vi "3.1.vi"() -> ()   [LabVIEW 2017]
panel:
  out "波形图":dbl[](graph)
  out "平均":dbl
  out "最小":dbl
  out "最大":dbl
  in  "长按停止":bool
  in  "生成随机数":bool
  # "任务一"
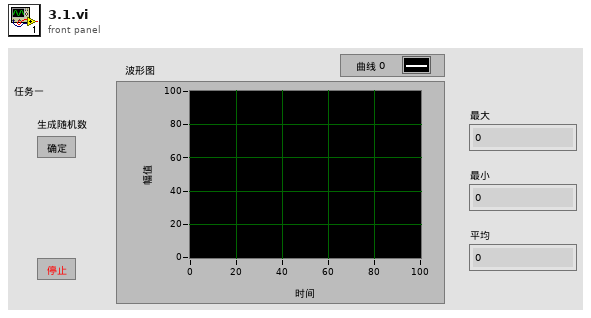
[diagram p1: front panel]
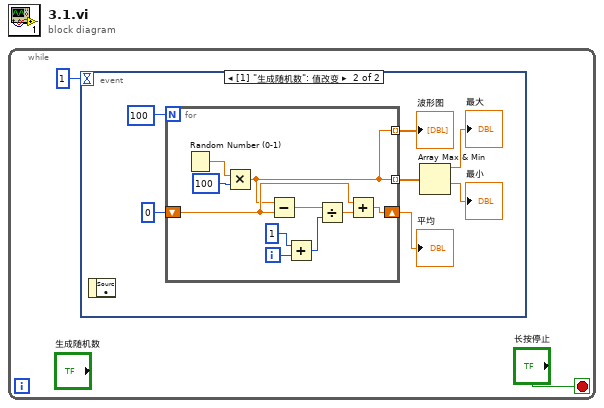
[diagram p0: block diagram]
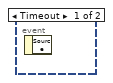
[diagram p2: hidden frame]
diagram:
  n1 = while {
    stop <- "长按停止" stop-if-true
    n2 = event shown="[1] \"生成随机数\": 值改变" {
      selector: _ -> [_ _]
      dyn-events: _ -> [_ _]
      timeout: 1 -> [_ _]
      event Timeout {
        n3 = event-data() -> ()  [unwired: 1 in, 1 out]
      }
      event "生成随机数": Value Change {
        n4 = event-data() -> ()  [unwired: 1 in, 1 out]
        n5 = for {
          N: 100 -> [_]
          tunnel: [w10] -> w8 mode=indexing
          shift-right: [w17] -> w4
          shift-left: 0 -> [w13]
          tunnel: [w10] -> w3 mode=indexing
          i -> [w18]
          n6 = Random Number (0-1)() -> (number: 0 to 1=w12:dbl)
          n7 = Multiply(x=w12, y=100) -> (x*y=w10:dbl)
          n8 = Subtract(x=w10, y=w13) -> (x-y=w16:dbl)
          n9 = Add(x=1, y=w18) -> (x+y=w15:i32)
          n10 = Divide(x=w16, y=w15) -> (x/y=w14:dbl)
          n11 = Add(x=w13, y=w14) -> (x+y=w17:dbl)
        }
        "平均" <- w4
        "波形图" <- w3
        n12 = Array Max & Min(array=w8) -> (max value=→"最大":dbl, min value=→"最小":dbl)  [unwired: 2 out]
      }
    }
  }
